vi "Auto Synch.vi"(8 "error in":errorcluster, 11 "Instrument Handle In":i32) -> (0 "error out":errorcluster, 3 "Instrument Handle Out":i32)   [LabVIEW 8.6, in "ZTScopeM.lvlib"]
doc: "Set the instrument to transfer the next successful capture to the auto download buffer."
uses:
  ZTScopeM.lvlib
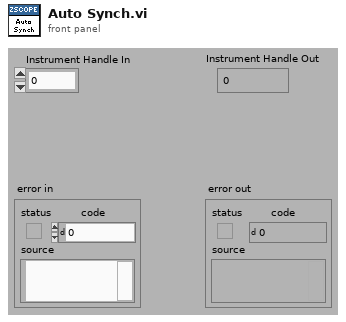
[diagram p1: front panel]
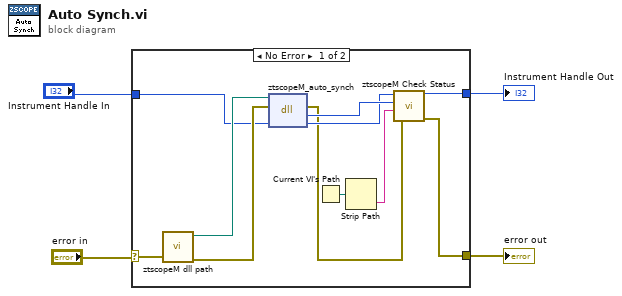
[diagram p0: block diagram]
diagram:
  n1 = case shown="No Error" "error in" {
    selector: "error in" -> [w9 w17]
    tunnel: [w10 w17] -> w3
    tunnel: [w11 w16] -> w2
    tunnel: "Instrument Handle In" -> [w5 w16]
    frame #0 {
      n2 = call "ztscopeM dll path.vi"("error in (no error)"=w9) -> ("error out"=w7:errorcluster, "<instrument>.dll path"=w8:path)  [unwired: 9 in]
      n3 = dll-call lib="C:/Program Files (x86)/National Instruments/LabVIEW 2013/instr.lib/ztscopem/ztscopeM.dll" fn="ztscopeM_auto_synch"(path in=w8, error in=w7, "instrumentHandle"=w5) -> (error out=w6:errorcluster, w15:i32, "instrumentHandle"=w14:i32)  [unwired: 1 in, 1 out]
      n4 = Current VI's Path() -> (path=w13:path)
      n5 = Strip Path(path=w13) -> (name=w12:string)  [unwired: 1 out]
      n6 = call "ztscopeM Check Status.vi"("error in"=w6, "name of VI"=w12, "status (return code)"=w15, "instrument handle in"=w14) -> ("error out"=w10:errorcluster, "instrument handle out"=w11:i32)  [unwired: 2 out]
    }
    frame #1 {
    }
  }
  "Instrument Handle Out" <- w2
  "error out" <- w3
